vi "GlobalFramesToStr.vi"() -> ()   [LabVIEW 2010]
panel:
  in  "Frames to Store":u32
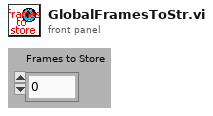
[diagram p1: front panel]
diagram:
